vi "parse_QuaternionStamped.vi"(4 "error in":errorcluster, 7 "msg in":string) -> (0 "error out":errorcluster, 2 "Quaternion":cluster{"x":dbl, "y":dbl, "z":dbl, "w":dbl}, 3 "msg out":string)   [LabVIEW 2012]
doc: "Parses a message into a quaternion stamped"
panel:
  out "Header":T1
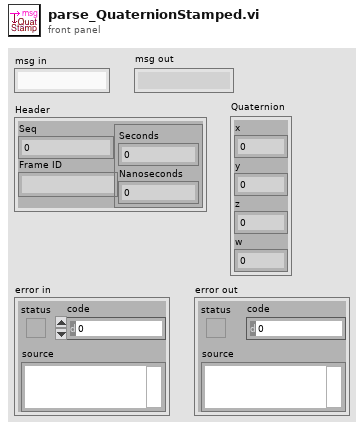
[diagram p1: front panel]
types:
  T1 = cluster{"Seq":u32, "Frame ID":string, "Timestamp":cluster{"Seconds":i32, "Nanoseconds":i32}}
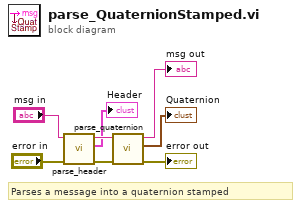
[diagram p0: block diagram]
diagram:
  # "Parses a message into a quaternion stamped"
  n1 = call <userlib>:"parse_header.vi"("error in"="error in", "msg in"="msg in") -> ("error out"=w1:errorcluster, "Header"=→"Header":T1, "msg out"=w3:string)  [unwired: 3 in]
  n2 = call <userlib>:"parse_quaternion.vi"("error in"=w1, "msg in"=w3) -> ("error out"=→"error out":errorcluster, "Quaternion"=→"Quaternion":cluster{"x":dbl, "y":dbl, "z":dbl, "w":dbl}, "msg out"=→"msg out":string)  [unwired: 3 in]
